vi "Check for Quit Condition.vi"() -> (3 "Quit?":bool)   [LabVIEW 2017]
uses:
  Global Variables.vi
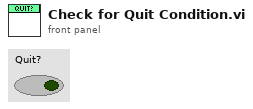
[diagram p1: front panel]
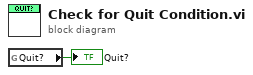
[diagram p0: block diagram]
diagram:
  n1 = global read "Global Variables.vi" "Quit?"() -> (→"Quit?":bool)
